vi "Step Counter.Inc Cnt and Append Prefix.vi"(10 "Section":string, 11 "Ctr":i32) -> (2 "Step ID":string, 3 "Ctr Out":i32)   [LabVIEW 2018]
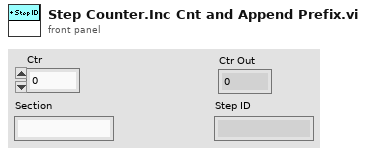
[diagram p1: front panel]
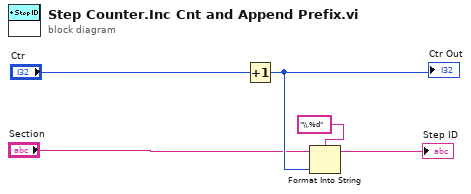
[diagram p0: block diagram]
diagram:
  n1 = Increment(x="Ctr") -> (x+1=w4:i32)
  "Ctr Out" <- w4
  n2 = Format Into String(format string="\\.%d", initial string="Section", w4) -> (resulting string=→"Step ID":string)  [unwired: 1 in, 1 out]
